vi "Populate Test DirectoryV3.vi"(8 "error in (no error)":errorcluster, 9 "FilePaths to Exclude":path[](array[path]), 10 "Main Folder Path":path, 11 "Study Tree (live)":refnum<vi>) -> (0 "error out":errorcluster)   [LabVIEW 2024]
uses:
  Modules/Tree Selection/Selection Global Method.ctl
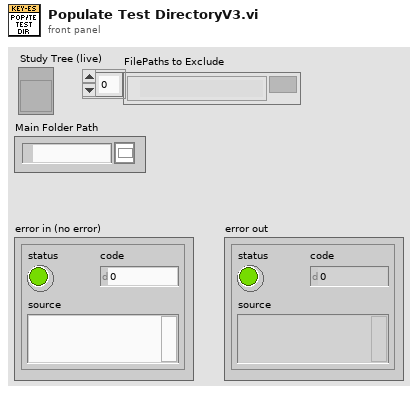
[diagram p1: front panel]
types:
  T1 = typedef "Selection Global Method.ctl" = enum16{"Read Selection", "Force Selection", "Mouse Down Event", "Select All", "Select None", "Invert Selection", "Read Selection and Tags"}
  T2 = cluster{"Left Cell String":string, "Child Text":string[], "Child Tag":string, "Item Indent":i32, "Child Only?":bool, "Glyph Index":i32}[]
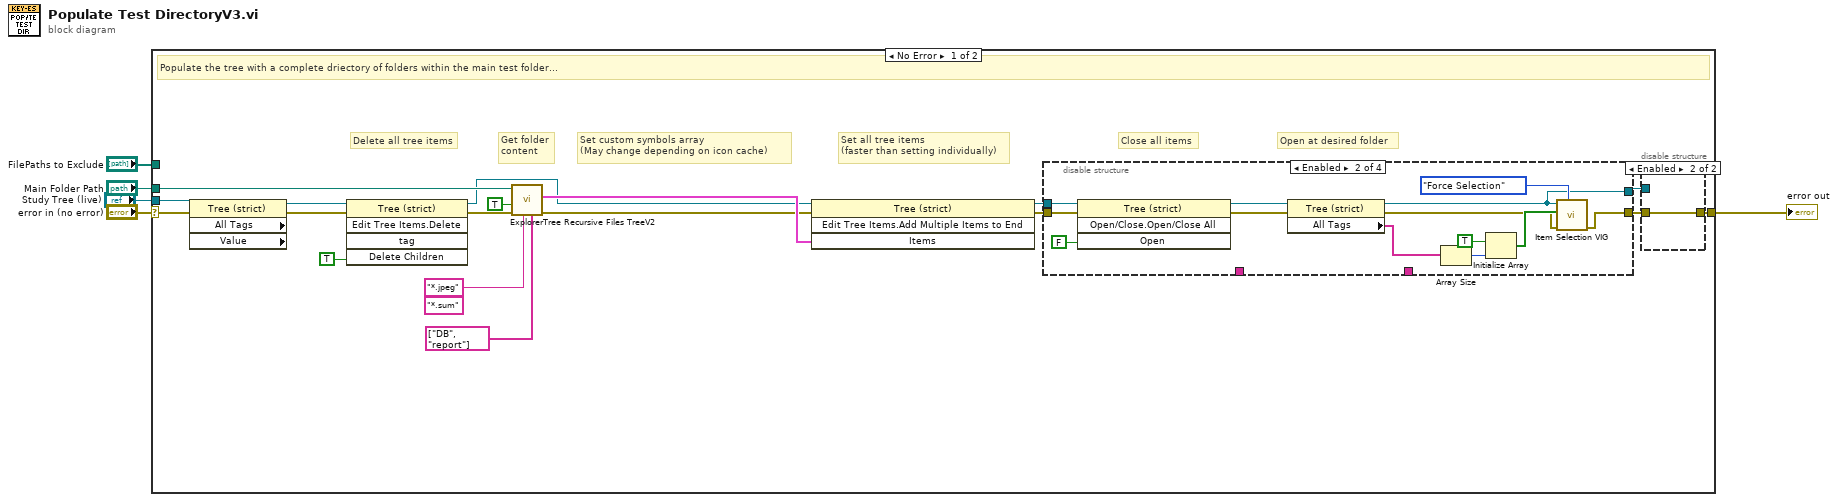
[diagram p0: block diagram]
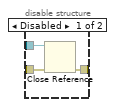
[diagram p2: hidden frame]
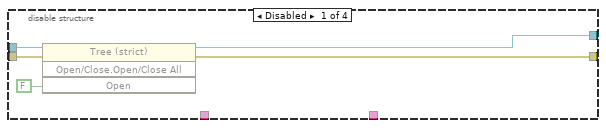
[diagram p3: hidden frame]
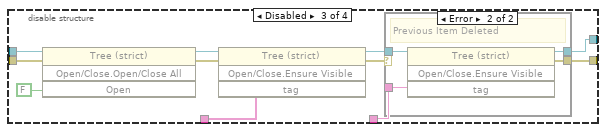
[diagram p4: hidden frame]
diagram:
  n1 = case shown="No Error" "error in (no error)" {
    selector: "error in (no error)" -> [w14 w64]
    tunnel: [w22 w64] -> w5
    tunnel: "Main Folder Path" -> [w15 _]
    tunnel: "FilePaths to Exclude" -> [_ _]
    tunnel: "Study Tree (live)" -> [w11 _]
    frame No Error {
      (unwired) "*.sum" ("Pattern")
      # "Open at desired folder"
      # "Close all items"
      # "Set all tree items\n(faster than setting individually)"
      # "Set custom symbols array\n(May change depending on icon cache)"
      # "Get folder\ncontent"
      # "Delete all tree items"
      # "Populate the tree with a complete driectory of folders within the main test folder..."
      n2 = property class="Tree (strict)" props=["All Tags", "Value"](reference=w11) -> (reference out=w13:refnum<vi>)  [unwired: 1 in, 3 out]
      n3 = invoke class="Tree (strict)" method="Edit Tree Items.Delete"(reference=w13, error in=w14, "Delete Children"=TRUE ("Delete Children?")) -> (reference out=w7:refnum<vi>, error out=w17:errorcluster)  [unwired: 2 in, 3 out]
      n4 = call "ExplorerTree Recursive Files TreeV2.vi"("Folders to Exclude"=string[] ["DB", "report"], "Pattern"="*.jpeg", "error in (no error)"=w17, "Continue Recursing on Error? (F)"=TRUE, "Folder Path"=w15) -> ("error out"=w6:errorcluster, "Items"=w9:T2)  [unwired: 3 in, 2 out]
      n5 = invoke class="Tree (strict)" method="Edit Tree Items.Add Multiple Items to End"(reference=w7, error in=w6, "Items"=w9) -> (reference out=w19:refnum<vi>, error out=w18:errorcluster)  [unwired: 1 in, 2 out]
      n6 = disable-structure shown="Enabled" {
        disable-tunnel: [w28 w32 w47 w62] -> w21
        disable-tunnel: [w27 w35 w48 w63] -> w20
        disable-tunnel: w19 -> [w30 w43 w52 w62]
        disable-tunnel: w18 -> [w29 w42 w51 w63]
        disable-tunnel: _ -> [_ _ w50 _]
        disable-tunnel: _ -> [_ _ w45 _]
        frame Disabled {
          n7 = invoke class="Tree (strict)" method="Open/Close.Open/Close All"(reference=w30, error in=w29, "Open"=FALSE ("Open?")) -> (reference out=w28:refnum<vi>, error out=w27:errorcluster)  [unwired: 1 in, 2 out]
        }
        frame Enabled {
          n8 = invoke class="Tree (strict)" method="Open/Close.Open/Close All"(reference=w43, error in=w42, "Open"=FALSE ("Open?")) -> (reference out=w36:refnum<vi>, error out=w34:errorcluster)  [unwired: 1 in, 2 out]
          n9 = property class="Tree (strict)"(reference=w36, error in=w34) -> (reference out=w32:refnum<vi>, error out=w33:errorcluster, "All Tags"=w41:string[])
          n10 = Array Size(array=w41) -> (size(s)=w39:i32)
          n11 = Initialize Array(TRUE, w39) -> (w40:bool[])
          n12 = call "Item Selection VIG.vi"("Method (Read Selection)"=Selection_Global_Method."Force Selection", "error in (no error)"=w33, "Selection"=w40, "Listbox or Tree"=w32) -> ("error out"=w35:errorcluster)  [unwired: 5 in, 2 out]
        }
        frame Disabled {
          n13 = invoke class="Tree (strict)" method="Open/Close.Open/Close All"(reference=w52, error in=w51, "Open"=FALSE ("Open?")) -> (reference out=w54:refnum<vi>, error out=w55:errorcluster)  [unwired: 1 in, 2 out]
          n14 = invoke class="Tree (strict)" method="Open/Close.Ensure Visible"(reference=w54, error in=w55, "tag"=w50) -> (reference out=w49:refnum<vi>, error out=w46:errorcluster)  [unwired: 1 in, 2 out]
          n15 = case shown="Error" w46 {
            selector: w46 -> [w57 _]
            tunnel: w49 -> [w56 w61]
            tunnel: [w57 w60] -> w48
            tunnel: [w56 w59] -> w47
            tunnel: w45 -> [_ w58]
            frame No Error {
            }
            frame Error {
              # "Previous Item Deleted"
              n16 = invoke class="Tree (strict)" method="Open/Close.Ensure Visible"(reference=w61, "tag"=w58) -> (reference out=w59:refnum<vi>, error out=w60:errorcluster)  [unwired: 2 in, 2 out]
            }
          }
        }
        frame Disabled {
        }
      }
      n17 = disable-structure shown="Enabled" {
        disable-tunnel: [w25 w26] -> w22
        disable-tunnel: w21 -> [w24 _]
        disable-tunnel: w20 -> [w23 w26]
        frame Disabled {
          n18 = Close Reference(reference=w24, error in (no error)=w23) -> (error out=w25:errorcluster)
        }
        frame Enabled {
        }
      }
    }
    frame Error {
    }
  }
  "error out" <- w5
